vi "去掉字符串空格.vi"(3 "含空格字符串":string) -> (0 "长度":i32, 1 "去掉空格字符串":string)   [LabVIEW 2016, in "数据传输系统-03.lvlib" / "自动更新.lvlib" / "TCP文件传输系统.lvlib" / "TCP发送文件.lvlib"]
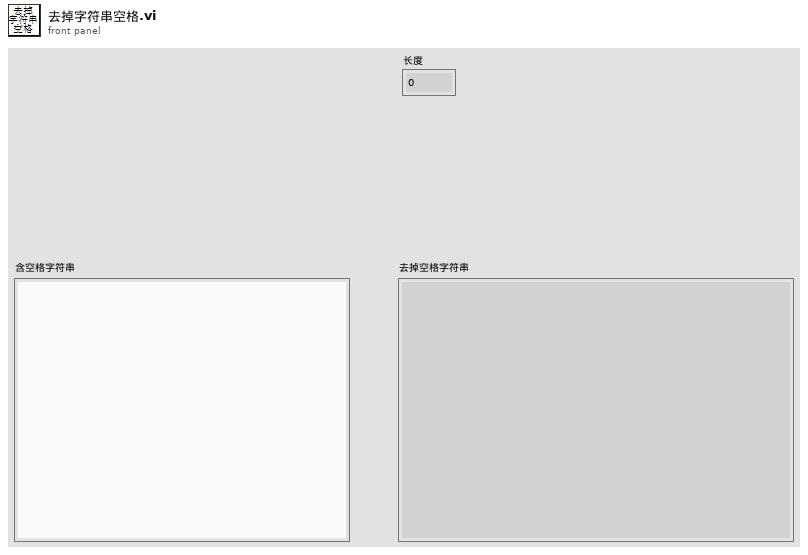
[diagram p1: front panel]
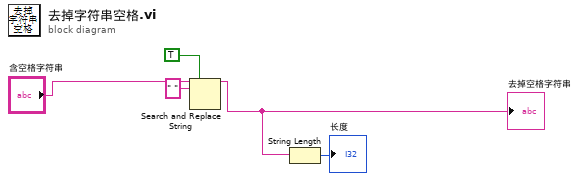
[diagram p0: block diagram]
diagram:
  n1 = Search and Replace String(replace all?=TRUE ("替换全部？(F)"), input string="含空格字符串", search string=" " ("搜索字符串")) -> (result string=w2:string)  [unwired: 5 in, 3 out]
  "去掉空格字符串" <- w2
  n2 = String Length(string=w2) -> (length=→"长度":i32)
